vi "Step Out.vi"(8 "error in (no error)":errorcluster, 11 "QUEUE in":refnum<queue>) -> (0 "error out":errorcluster, 1 "elements":cluster{"State":string, "Data":variant}[](array[cluster]), 2 "element":cluster{"State":string, "Data":variant}={"State"="GUI::Display", "Data"=variant}, 3 "queue out":refnum<queue>)   [LabVIEW 2016]
panel:
  out "# elements in queue":i32
  out "max queue size":i32
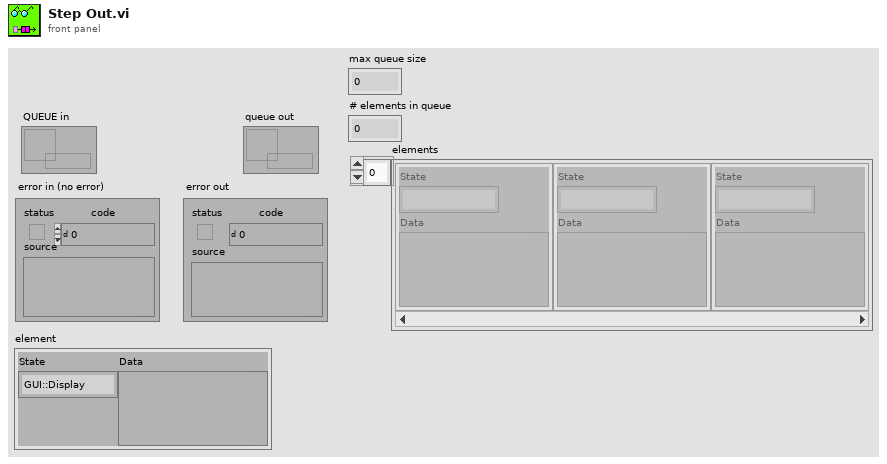
[diagram p1: front panel]
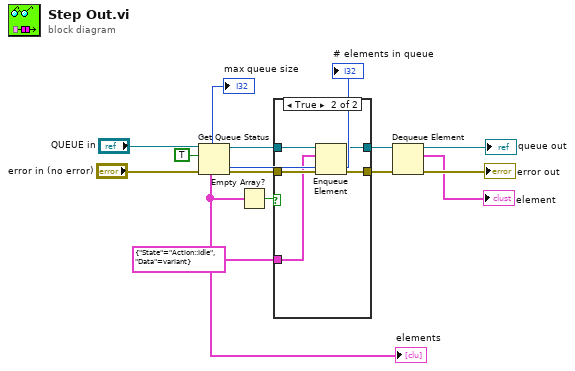
[diagram p0: block diagram]
diagram:
  n1 = Get Queue Status(queue="QUEUE in", return elements? (F)=TRUE, error in (no error)="error in (no error)") -> (queue out=w11:refnum<queue>, max queue size=→"max queue size":i32, error out=w9:errorcluster, # elements in queue=→"# elements in queue":i32, elements=w13:cluster{"State":string, "Data":variant}[])  [unwired: 3 out]
  "elements" <- w13
  n2 = Empty Array?(array=w13) -> (empty?=w12:bool)
  n3 = case shown="True" w12 {
    tunnel: w11 -> [w17 w22]
    tunnel: [w17 w21] -> w10
    tunnel: w9 -> [w16 w20]
    tunnel: [w16 w19] -> w5
    tunnel: cluster{"State":string, "Data":variant} {"State"="Action::Idle", "Data"=variant} ("element") -> [_ w18]
    frame False {
    }
    frame True {
      n4 = Enqueue Element(queue=w22, element=w18, error in (no error)=w20) -> (queue out=w21:refnum<queue>, error out=w19:errorcluster)  [unwired: 1 in, 1 out]
    }
  }
  n5 = Dequeue Element(queue=w10, error in (no error)=w5) -> (queue out=→"queue out":refnum<queue>, element=→"element":cluster{"State":string, "Data":variant}, error out=→"error out":errorcluster)  [unwired: 1 in, 1 out]
